vi "PH_Img_BaseClass.ProcCases.vi"(0 "i ref in":refnum<vi>, 1 "selector":string, 2 "Data":T1, 3 "call cluster":T2={"Object"="", "Selector"="", "CallType"=enum."synchronous", "Async Object"="", "Async Selector"="", "Data Descriptor"="", "Data"=[], "Error #"=0, "Expire"=0}, 5 "error in (no error)":errorcluster) -> (14 "i ref out":refnum<vi>, 17 "answer cluster":T2={"Object"="", "Selector"="", "CallType"=enum."synchronous", "Async Object"="", "Async Selector"="", "Data Descriptor"="", "Data"=[], "Error #"=0, "Expire"=0}, 19 "error out":errorcluster)   [LabVIEW 2014, in "PH_Img_BaseClass.lvlib"]
doc: "This method is called by a process from within the default case in the event loop. The methods of a class that are linked to events will be called from THIS method. Add your code here."
uses:
  PH_Img_BaseClass.lvlib
  CSCore/CSSystem/CoreDefs/CoreDefs.call_type.ctl
  CSCore/BaseProcess/BaseProcess.descriptor string definition.ctl
  CSCore/CSSystem/CoreDefs/CoreDefs.rawDataType.ctl
  CSCore/CSSystem/CoreLib/CoreLib.string 2 byte array.vi
  CSCore/CSSystem/CoreLib/CoreLib.byte array 2 int.vi
  CSCore/BaseProcess/BaseProcess.lvlib
  CSCore/CSSystem/CoreLib/CoreLib.lvlib
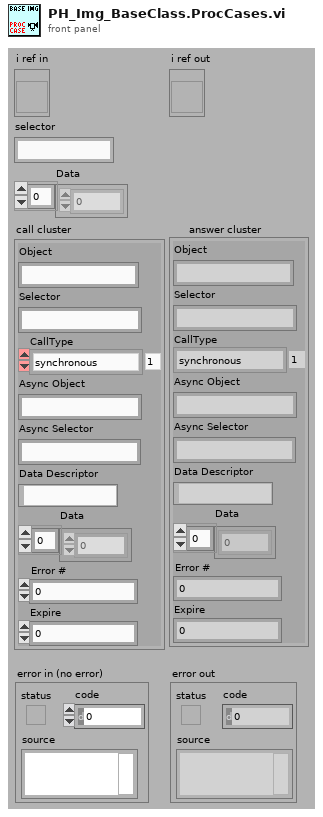
[diagram p1: front panel]
types:
  T1 = typedef "CoreDefs.rawDataType.ctl" = i8[]
  T2 = typedef "CoreDefs.call_type.ctl" = cluster{"Object":string, "Selector":string, "CallType":enum16{"simple", "synchronous", "asynchronous"}, "Async Object":string, "Async Selector":string, "Data Descriptor":T3, "Data":T1, "Error #":i32, "Expire":u32}
  T3 = typedef "BaseProcess.lvlib/BaseProcess.descriptor string definition.ctl" = string
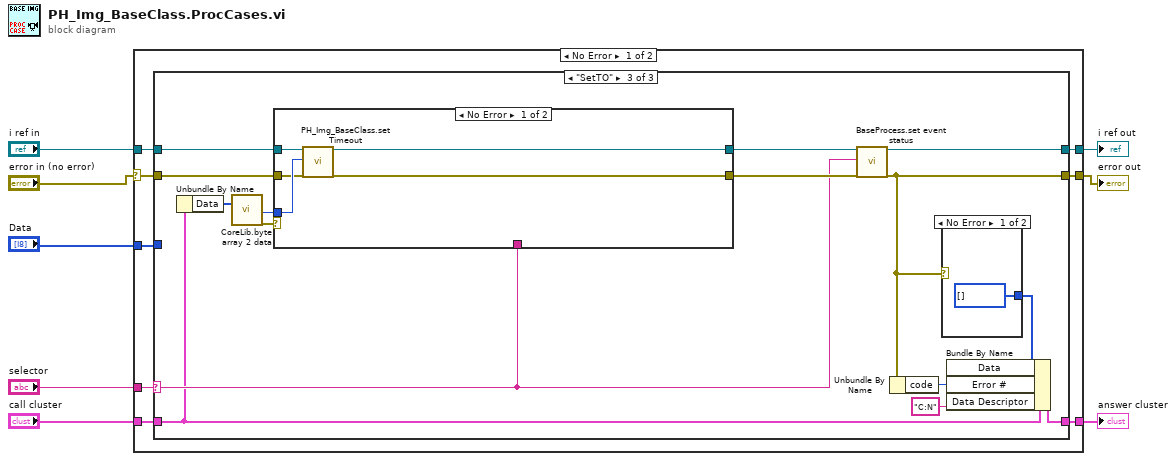
[diagram p0: block diagram]
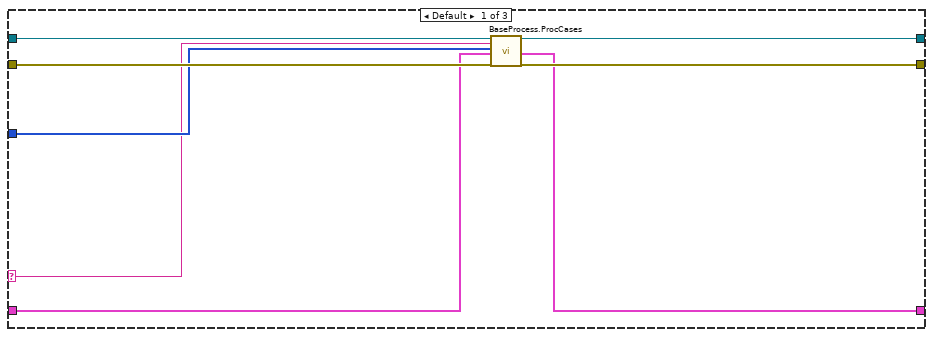
[diagram p2: hidden frame]
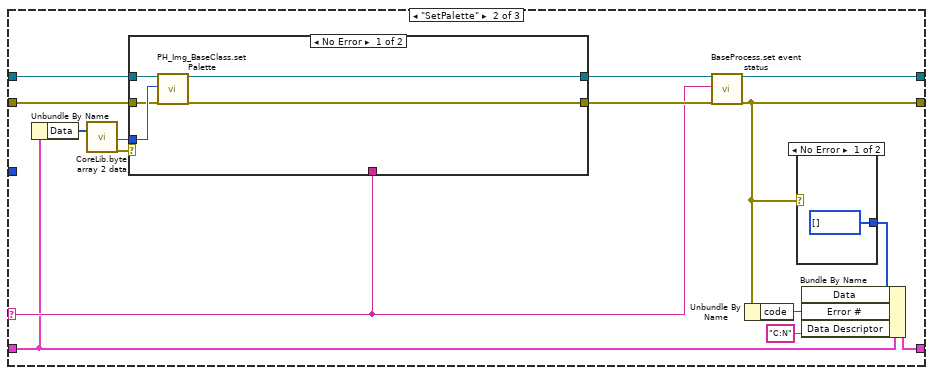
[diagram p3: hidden frame]
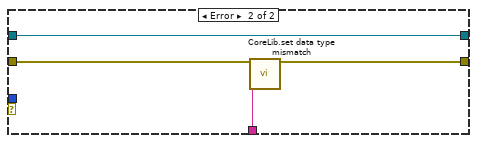
[diagram p4: hidden frame]
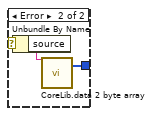
[diagram p5: hidden frame]
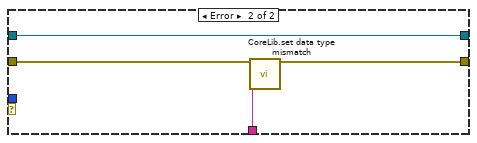
[diagram p6: hidden frame]
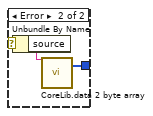
[diagram p7: hidden frame]
diagram:
  n1 = case shown="No Error" "error in (no error)" {
    selector: "error in (no error)" -> [w9 w81]
    tunnel: "selector" -> [w16 _]
    tunnel: [w15 w82] -> w7
    tunnel: "Data" -> [w14 _]
    tunnel: "call cluster" -> [w13 w82]
    tunnel: "i ref in" -> [w12 w83]
    tunnel: [w11 w83] -> w3
    tunnel: [w10 w81] -> w2
    frame No Error {
      n2 = case shown="\"SetTO\"" w16 {
        selector: w16 -> [w18 w27 w55]
        tunnel: w14 -> [w19 _ _]
        tunnel: w12 -> [w17 w31 w59]
        tunnel: [w24 w29 w57] -> w11
        tunnel: w13 -> [w20 w26 w54]
        tunnel: [w21 w25 w53] -> w15
        tunnel: w9 -> [w23 w30 w58]
        tunnel: [w22 w28 w56] -> w10
        frame Default {
          n3 = call "BaseProcess.ProcCases.vi"("i ref in"=w17, "selector"=w18, "Data"=w19, "call cluster"=w20, "error in (no error)"=w23) -> ("i ref out"=w24:refnum<vi>, "answer cluster"=w21:T2, "error out"=w22:errorcluster)  [unwired: 12 in]
        }
        frame "SetPalette" {
          n4 = Unbundle By Name(w26) -> ("Data"=w36:T1)
          n5 = call-poly "CoreLib.byte array 2 data.vi"("byteArray"=w36) -> ("i32"=w34:i32, "error out"=w35:errorcluster)  [unwired: 16 in, 1 out]
          n6 = case shown="No Error" w35 {
            tunnel: [w44 w48] -> w32
            tunnel: w31 -> [w40 w48]
            tunnel: w30 -> [w41 w47]
            tunnel: [w43 w46] -> w33
            tunnel: w34 -> [w42 _]
            tunnel: w27 -> [_ w45]
            frame No Error {
              n7 = call "PH_Img_BaseClass.set Palette.vi"("i ref in"=w40, "Palette"=w42, "error in (no error)"=w41) -> ("i ref out"=w44:refnum<vi>, "error out"=w43:errorcluster)  [unwired: 15 in]
            }
            frame Error {
              n8 = call "CoreLib.set data type mismatch.vi"("error in (no error)"=w47, "error source"=w45) -> ("error out"=w46:errorcluster)  [unwired: 17 in]
            }
          }
          n9 = call "BaseProcess.set event status.vi"("i ref in"=w32, "EventStatus"=w27, "error in (no error)"=w33) -> ("i ref out"=w29:refnum<vi>, "error out"=w28:errorcluster)  [unwired: 14 in, 1 out]
          n10 = Unbundle By Name(w28) -> ("code"=w39:i32)
          n11 = case shown="No Error" w28 {
            selector: w28 -> [_ w52]
            tunnel: [T1 [] ("byteArray out") w51] -> w38
            frame No Error {
            }
            frame Error {
              n12 = Unbundle By Name(w52) -> ("source"=w50:string)
              n13 = call-poly "CoreLib.data 2 byte array.vi"("string"=w50) -> ("byteArray out"=w51:T1)  [unwired: 18 in]
            }
          }
          n14 = Bundle By Name(cluster=w26, "Data"=w38, "Error #"=w39, "Data Descriptor"="C:N") -> (w25:T2)
        }
        frame "SetTO" {
          n15 = Unbundle By Name(w54) -> ("Data"=w64:T1)
          n16 = call-poly "CoreLib.byte array 2 data.vi"("byteArray"=w64) -> ("i32"=w62:i32, "error out"=w63:errorcluster)  [unwired: 16 in, 1 out]
          n17 = case shown="No Error" w63 {
            tunnel: [w72 w76] -> w60
            tunnel: w59 -> [w68 w76]
            tunnel: w58 -> [w69 w75]
            tunnel: [w71 w74] -> w61
            tunnel: w62 -> [w70 _]
            tunnel: w55 -> [_ w73]
            frame No Error {
              n18 = call "PH_Img_BaseClass.set Timeout.vi"("i ref in"=w68, "Timeout Image [ms]"=w70, "error in (no error)"=w69) -> ("i ref out"=w72:refnum<vi>, "error out"=w71:errorcluster)  [unwired: 15 in]
            }
            frame Error {
              n19 = call "CoreLib.set data type mismatch.vi"("error in (no error)"=w75, "error source"=w73) -> ("error out"=w74:errorcluster)  [unwired: 17 in]
            }
          }
          n20 = call "BaseProcess.set event status.vi"("i ref in"=w60, "EventStatus"=w55, "error in (no error)"=w61) -> ("i ref out"=w57:refnum<vi>, "error out"=w56:errorcluster)  [unwired: 14 in, 1 out]
          n21 = Unbundle By Name(w56) -> ("code"=w67:i32)
          n22 = case shown="No Error" w56 {
            selector: w56 -> [_ w80]
            tunnel: [T1 [] ("byteArray out") w79] -> w66
            frame No Error {
            }
            frame Error {
              n23 = Unbundle By Name(w80) -> ("source"=w78:string)
              n24 = call-poly "CoreLib.data 2 byte array.vi"("string"=w78) -> ("byteArray out"=w79:T1)  [unwired: 18 in]
            }
          }
          n25 = Bundle By Name(cluster=w54, "Data"=w66, "Error #"=w67, "Data Descriptor"="C:N") -> (w53:T2)
        }
      }
    }
    frame Error {
    }
  }
  "answer cluster" <- w7
  "i ref out" <- w3
  "error out" <- w2
